vi "HardwareConfiguration.vi"() -> (3 "configured?":bool)   [LabVIEW 2019]
uses:
  InstrControl/InstrumentSetup.vi
  globals/QC_RunInformation.vi
  InstrControl/InstrControl.lvclass
panel:
  in  "Matrix Configurations":bool
  in  "Defaults Multimeter":bool
  in  "Multimeter":enum32{"Keithley 2000"}(tab)
  in  "Range Value\n(0.1 - 100)":dbl=100.0 format="%#.2g"
  in  "Range":u16(ring) items=["Auto", "Manual"]
  in  "Function":u16(ring)=3 items=["AC Current", "DC Current", "AC Voltage", "DC Voltage", "2W-Resistance", "4W-Resistance", "Period", "Frequency", "Temperature", "Diode", "Continuity"]
  in  "GPIB Address KE2000":refnum<visa-resource-name>
  in  "Defaults LCR":bool
  in  "LCRs":enum32{"WayneKerr 6440B", "WayneKerr 6425"}(tab)
  in  "AC frequency [Hz]":i32=1000 format="%#.3p"
  in  "RC Configuration":u16(ring) items=["serial", "parallel"]
  in  "AC amplitude [V]":sgl=0.1
  in  "GPIB Address WK6440B":refnum<visa-resource-name>
  in  "GPIB Address WK6425":refnum<visa-resource-name>
  in  "AC amplitude [V] WK6425":sgl=0.1 caption="AC amplitude [V]"
  in  "RC Configuration WK6425":u16(ring) caption="RC Configuration" items=["serial", "parallel"]
  in  "AC frequency [Hz] WK6425":i32=1000 caption="AC frequency [Hz]" format="%#.3p"
  in  "VISA address":refnum<visa-resource-name>="COM24" caption="Arduino address"
  out "Programm uploaded?":string="Make sure programme is uploaded to Arduino Uno ->"
  in  "Blank Button":bool
  in  "Supplies":T1(tab)
  in  "Current Limit [µA]":sgl=100.0
  in  "GPIB Address KE2410":refnum<visa-resource-name>
  in  "2657A Current Limit [µA]":sgl=100.0 caption="Current Limit [µA]"
  in  "GPIB Address 2657A":refnum<visa-resource-name>
  in  "GPIB Address KE487":refnum<visa-resource-name>
  in  "Compliance":u16(ring) items=["20µA", "2mA"]
  in  "Range:":u16(ring) items=["Autorange", "2nA", "20nA", "200nA", "2 microAmp", "20 microAmp", "200 microAmp", "2 milliAmp"]
  in  "Current Limit":u16(ring)=1 items=["OFF", "ON"]
  in  "GPIB Address KE6517":refnum<visa-resource-name>
  in  "current compliance \nlevel [mA]":dbl=0.0001 format="%.4f"
  in  "compliance/measurement\nrange (auto:0)":u16(ring)=6 items=["auto / auto", "1 nA / 1.1 V", "10 nA / 11 V", "100 nA / 110 V", "0.001 mA / 110 V", "0.01 mA / 110 V", "0.1 mA / 110 V", "1 mA / 110 V", "10 mA / 110 V", "100 mA / 110 V"]
  in  "GPIB Address KE236":refnum<visa-resource-name>
  in  "Defaults Supply":bool
  in  "OK Button":bool
  # "Hardware Configuration"
  # "Multimeter Configuration"
  # "Supply Configuration"
  # "Arduino Configuration"
  # "LCR Configuration"
  # "(Only for initialisation)"
  # "(Only for initialisation)"
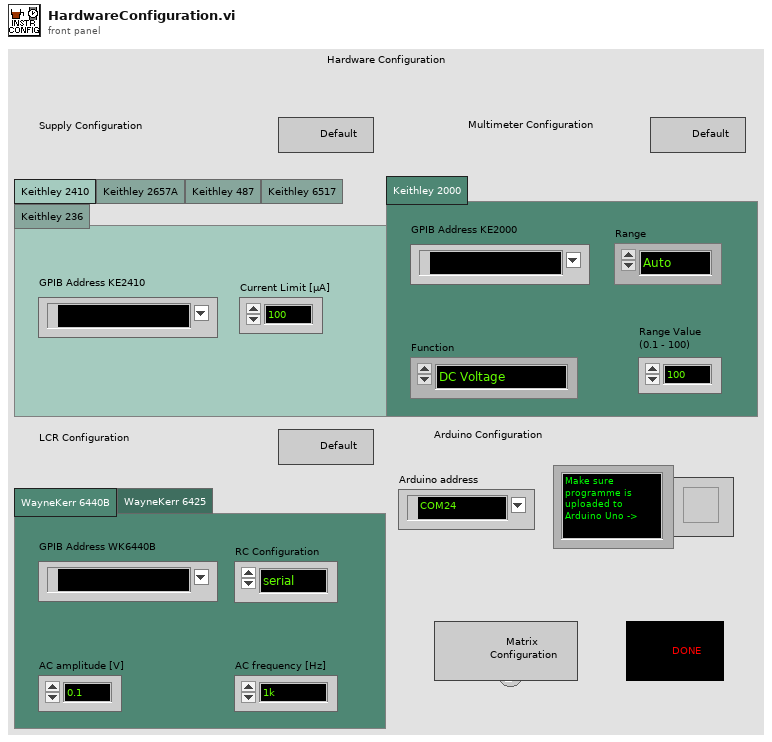
[diagram p1: front panel]
types:
  T1 = enum32{"Keithley 2410", "Keithley 2657A", "Keithley 487", "Keithley 6517", "Keithley 236"}
  T2 = cluster{"KE 2410":cluster{"Instrument name":string, "address":refnum<visa-resource-name>, "Instrument type":u16}, "KE 6517":cluster{"Instrument name":string, "address":refnum<visa-resource-name>, "Instrument type":u16}, "KE 487":cluster{"Instrument name":string, "address":refnum<visa-resource-name>, "Instrument type":u16}, "KE 236":cluster{"Instrument name":string, "address":refnum<visa-resource-name>, "Instrument type":u16}, "WK 6440B":cluster{"Instrument name":string, "address":refnum<visa-resource-name>, "Instrument type":u16}, "WK 6425":cluster{"Instrument name":string, "address":refnum<visa-resource-name>, "Instrument type":u16}, "Pickering Matrix":cluster{"Instrument name":string, "address":refnum<visa-resource-name>, "Instrument type":u16}, "KE 2000":cluster{"Instrument name":string, "address":refnum<visa-resource-name>, "Instrument type":u16}, "KE3706A Switching":cluster{"Instrument name":string, "address":refnum<visa-resource-name>, "Instrument type":u16}, "KE 2657A":cluster{"Instrument name":string, "address":refnum<visa-resource-name>, "Instrument type":u16}, "R_METAL KE2410":cluster{"Instrument name":string, "address":refnum<visa-resource-name>, "Instrument type":u16}, "HP34401A":cluster{"Instrument name":string, "address":refnum<visa-resource-name>, "Instrument type":u16}}
  T3 = cluster{"VISA address":refnum<visa-resource-name>, "T sensor":enum16{"SHT", "DS"}, "Arduino":refnum<class "ArduinoControl.lvclass">}
  T4 = cluster{"Range":u16, "Range Value":dbl, "Function":u16, "KE2000":refnum<class "KE2000.lvclass">}
  T5 = cluster{"Current Limit":sgl, "KE2410":refnum<class "KE2410.lvclass">}
  T6 = cluster{"Compliance":u16, "Range:":u16, "KE487":refnum<class "KE487.lvclass">}
  T7 = cluster{"Current Limit":sgl, "KE2657A":refnum<class "KE2657A.lvclass">}
  T8 = cluster{"Current Limit":u16, "KE6517":refnum<class "KE6517.lvclass">}
  T9 = cluster{"current \ncompliance level":dbl, "compliance/\nmeasurement range (auto:0)":u16, "KE236":refnum<class "KE236.lvclass">}
  T10 = cluster{"Sensor Serial No.:":string, "Wafer Serial No.:":string, "Batch:":string, "Manufacturer:":string, "Device Category:":string, "Database Serial No.:":string, "Date Initiated:":string, "Time Initiated:":string, "Test":string, "Instruments used:":string, "Probeplan used:":string, "End of Run comment:":string, "User:":string}
  T11 = cluster{"RC Configuration":u16, "AC amplitude [V]":dbl, "AC frequency [Hz]":i32, "WK6440B":refnum<class "WK6440B.lvclass">}
  T12 = cluster{"RC Configuration":u16, "AC amplitude [V]":dbl, "AC frequency [Hz]":i32, "WK6425":refnum<class "WK6425.lvclass">}
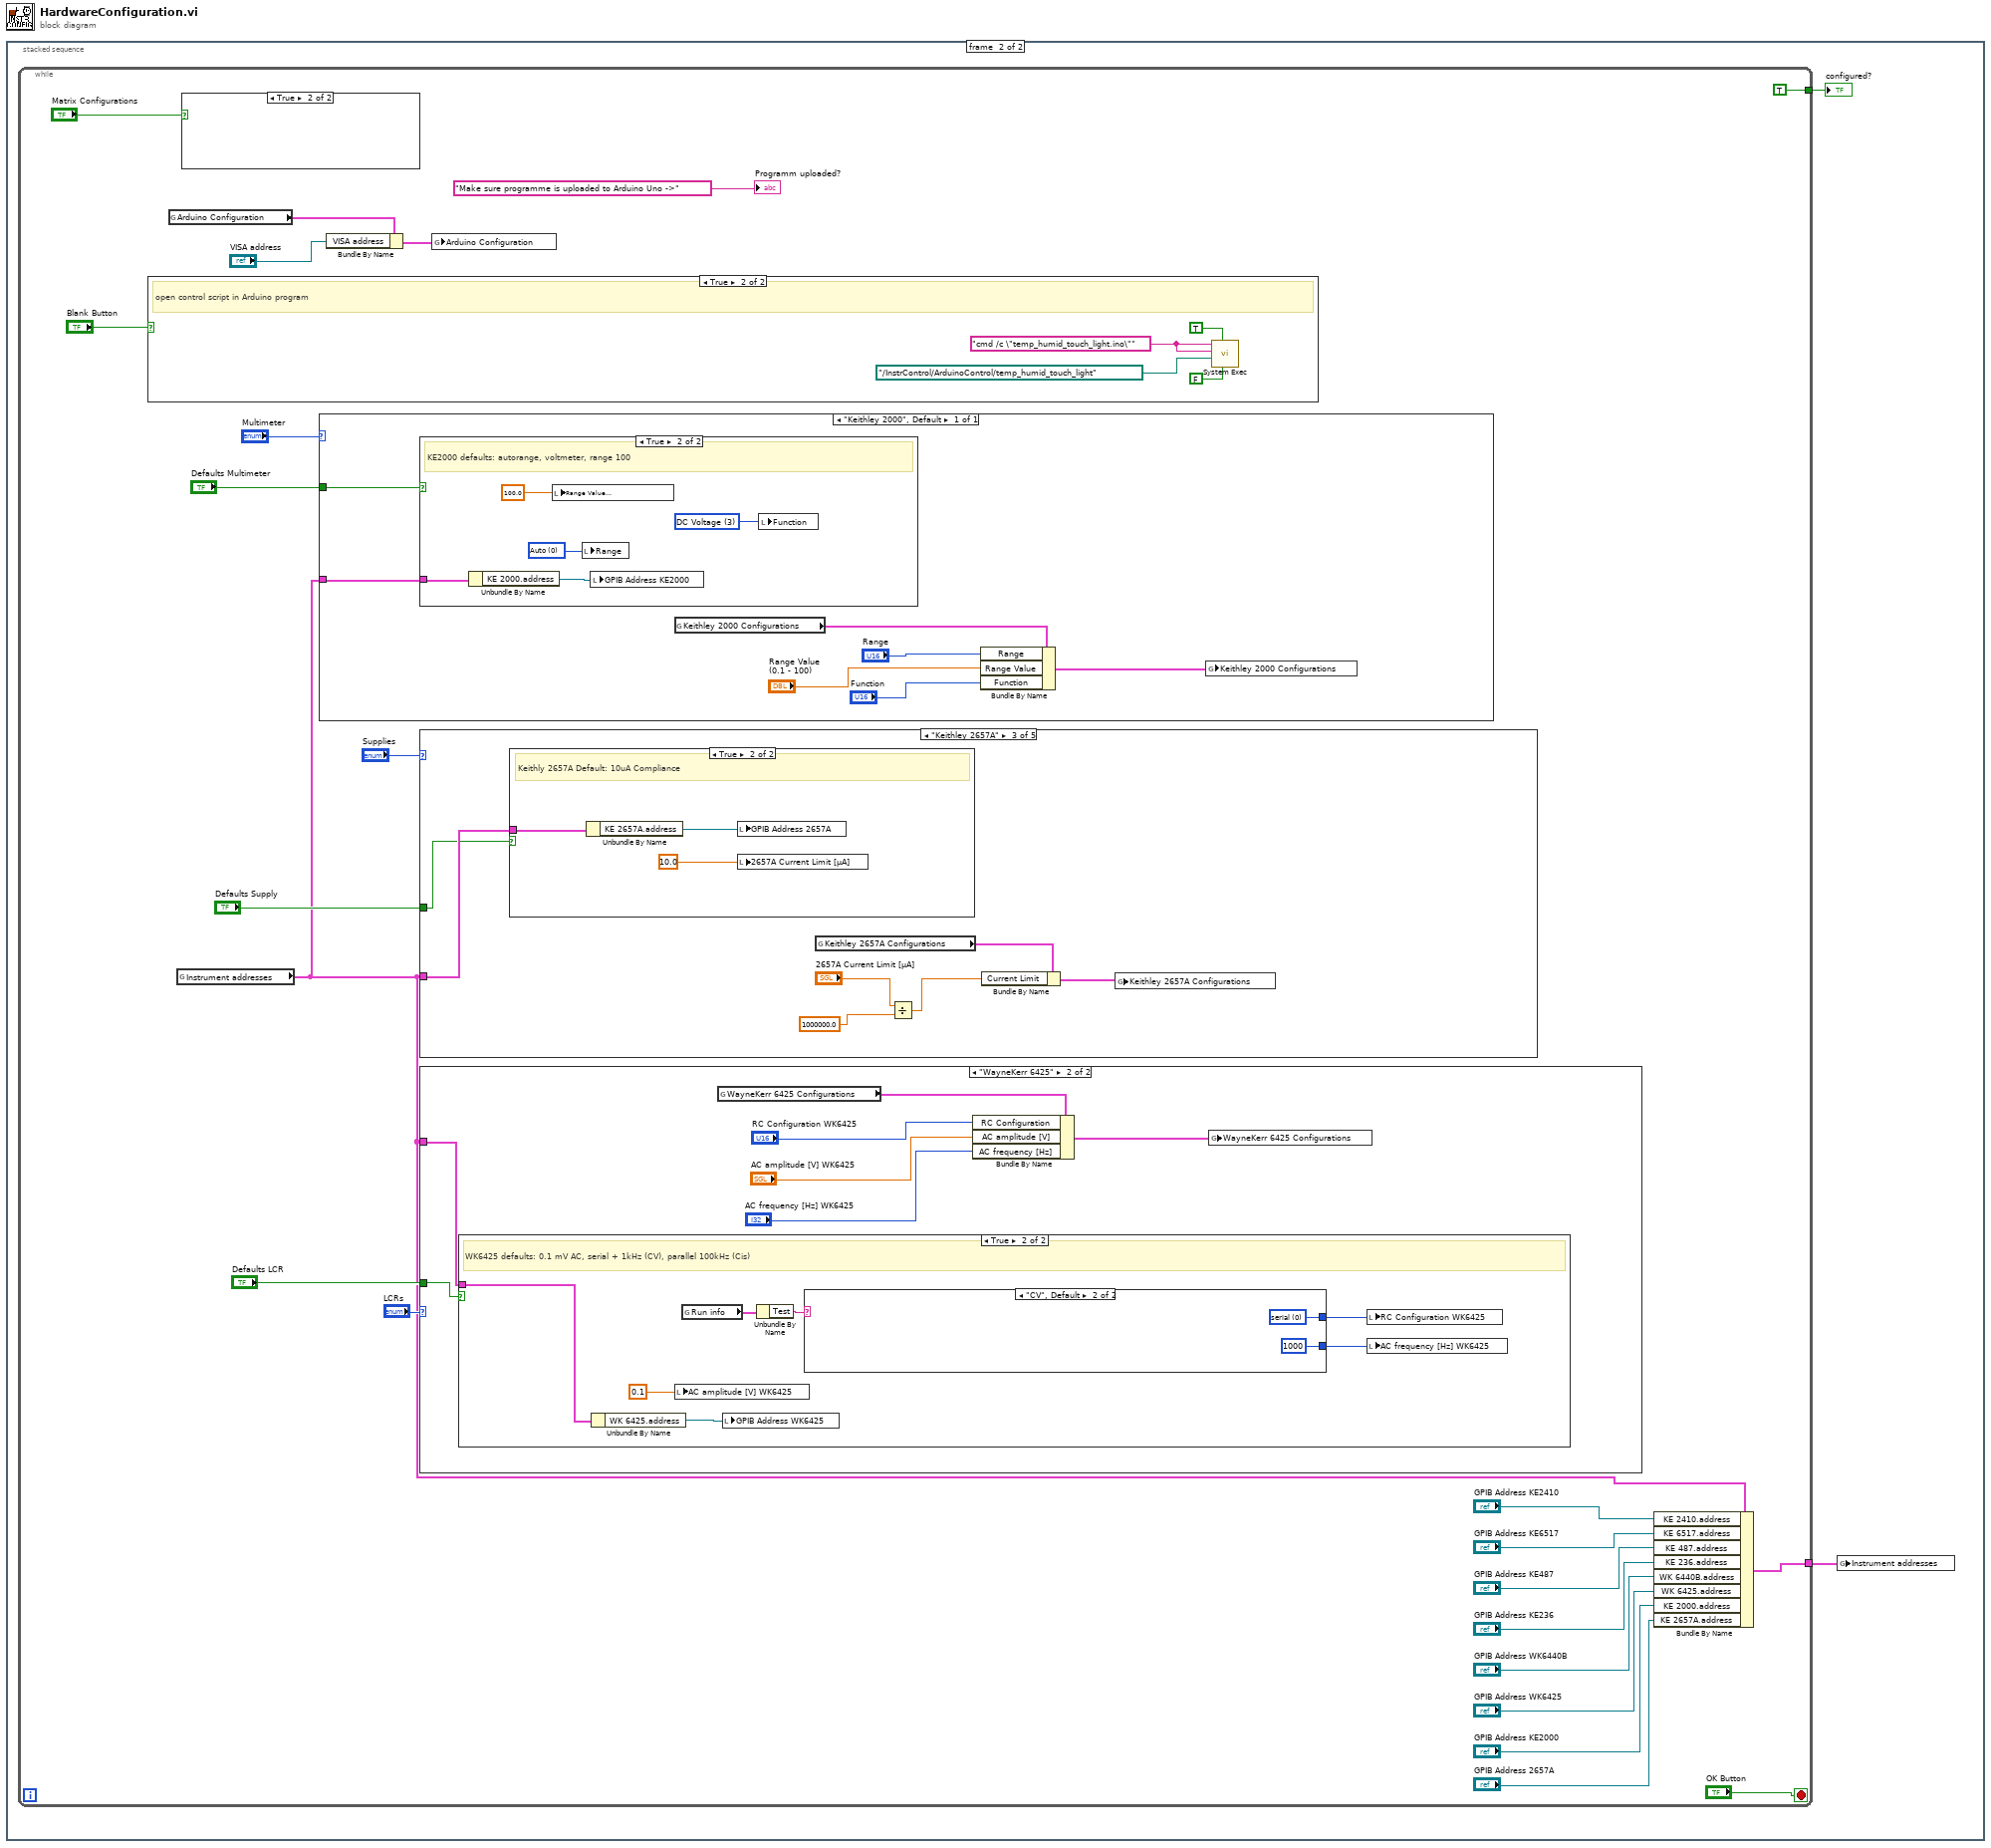
[diagram p0: block diagram]
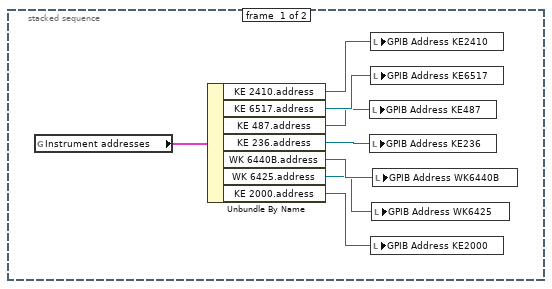
[diagram p2: hidden frame]
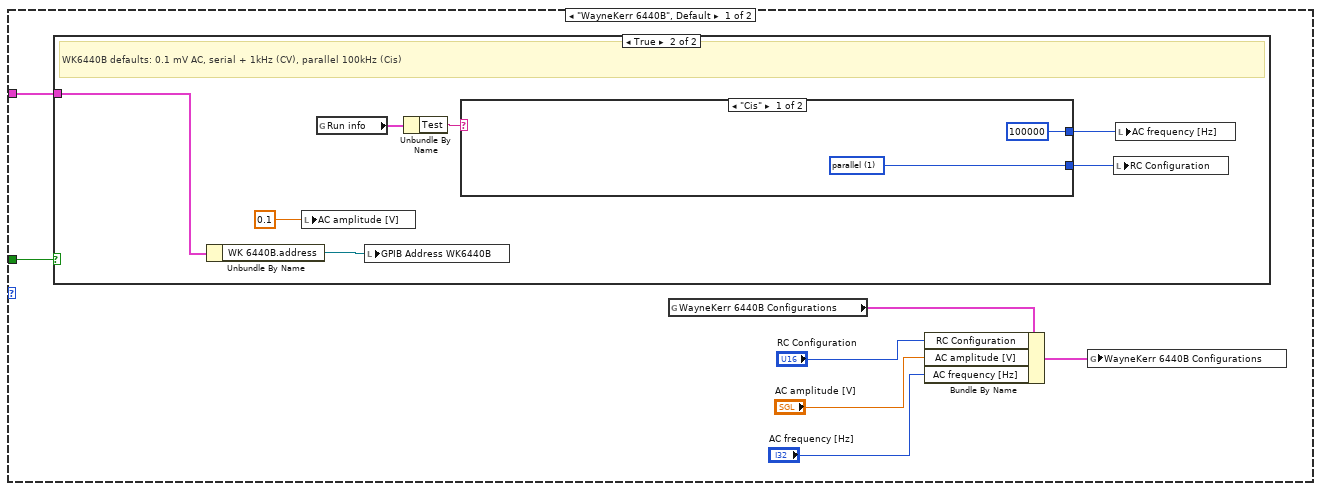
[diagram p6: hidden frame]
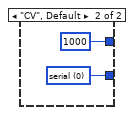
[diagram p8: hidden frame]
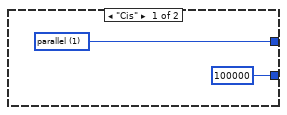
[diagram p10: hidden frame]
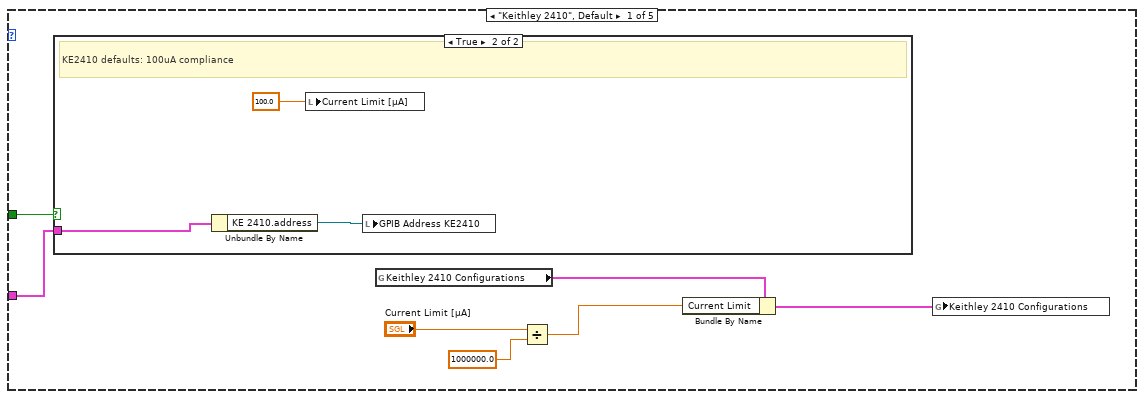
[diagram p11: hidden frame]
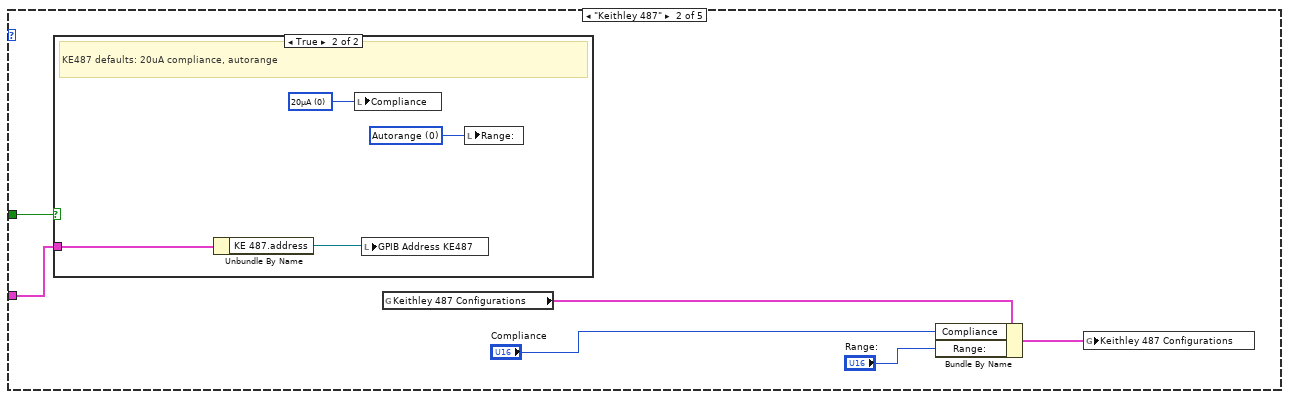
[diagram p13: hidden frame]
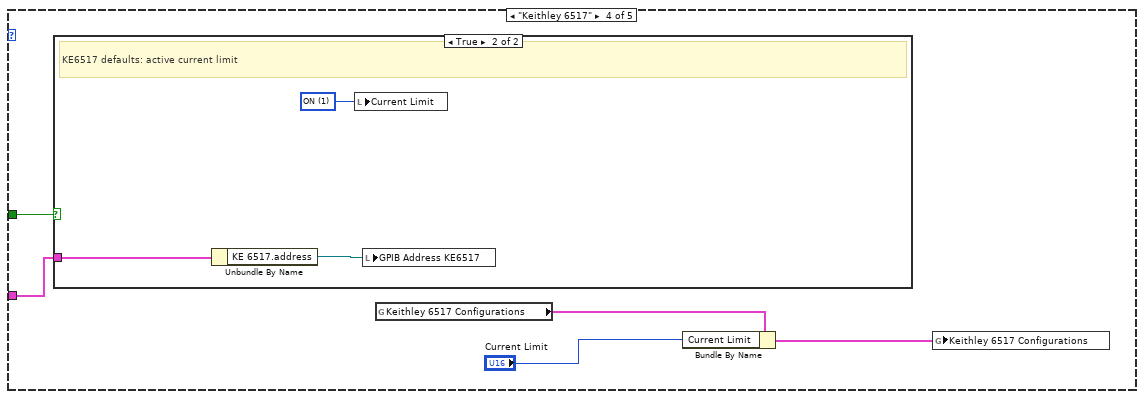
[diagram p16: hidden frame]
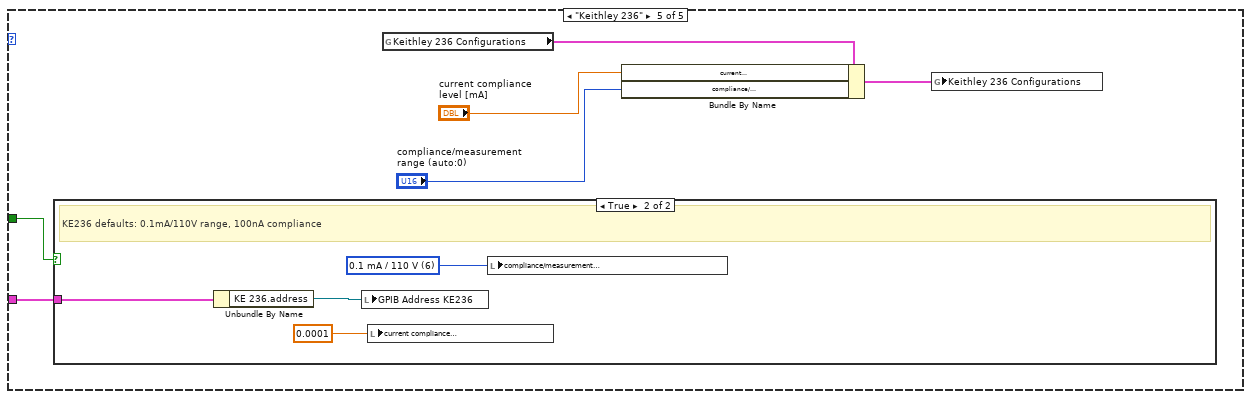
[diagram p18: hidden frame]
diagram:
  n1 = stacked-sequence {
    frame #0 {
      n2 = global read "InstrumentSetup.vi" "Instrument addresses"() -> (w8:T2)
      n3 = Unbundle By Name(w8) -> ("KE 2410.address"=w7:refnum<visa-resource-name>, "KE 6517.address"=w6:refnum<visa-resource-name>, "KE 487.address"=w5:refnum<visa-resource-name>, "KE 236.address"=w4:refnum<visa-resource-name>, "WK 6440B.address"=w3:refnum<visa-resource-name>, "WK 6425.address"=w2:refnum<visa-resource-name>, "KE 2000.address"=w1:refnum<visa-resource-name>)
      n4 = local write "GPIB Address KE487"(w5) -> ()
      n5 = local write "GPIB Address KE236"(w4) -> ()
      n6 = local write "GPIB Address KE2410"(w7) -> ()
      n7 = local write "GPIB Address KE6517"(w6) -> ()
      n8 = local write "GPIB Address KE2000"(w1) -> ()
      n9 = local write "GPIB Address WK6425"(w2) -> ()
      n10 = local write "GPIB Address WK6440B"(w3) -> ()
    }
    frame #1 {
      n11 = while {
        tunnel: [TRUE] -> w10
        tunnel: [w18] -> w9
        stop <- "OK Button" stop-if-true
        n12 = case shown="True" "Blank Button" {
          frame False {
          }
          frame True {
            w36 = "cmd /c \"temp_humid_touch_light.ino\""
            # "open control script in Arduino program"
            n13 = call <vilib>:"System Exec.vi"("run minimized? (F)"=FALSE, "wait until completion? (T)"=TRUE, "working directory"=path "../InstrControl/ArduinoControl/temp_humid_touch_light", "standard input"=w36, "command line"=w36) -> ()  [unwired: 3 in, 4 out]
          }
        }
        n14 = global read "InstrumentSetup.vi" "Arduino Configuration"() -> (w25:T3)
        n15 = global read "InstrumentSetup.vi" "Instrument addresses"() -> (w20:T2)
        n16 = case shown="True" "Matrix Configurations" {
          frame False {
          }
          frame True {
          }
        }
        n17 = case shown="\"Keithley 2000\", Default" "Multimeter" {
          tunnel: "Defaults Multimeter" -> [w45]
          tunnel: w20 -> [w42]
          frame "Keithley 2000", Default {
            n18 = case shown="True" w45 {
              tunnel: w42 -> [_ w50]
              frame False {
              }
              frame True {
                w48 = u16 0 items=["Auto", "Manual"] ("Range")
                w49 = u16 3 items=["AC Current", "DC Current", "AC Voltage", "DC Voltage", "2W-Resistance", "4W-Resistance", "Period", "Frequency", "Temperature", "Diode", "Continuity"] ("Function")
                # "KE2000 defaults: autorange, voltmeter, range 100"
                n19 = Unbundle By Name(w50) -> ("KE 2000.address"=w46:refnum<visa-resource-name>)
                n20 = local write "Range Value\n(0.1 - 100)"(100.0 ("Range Value\n(0.1 - 100)")) -> ()
                n21 = local write "Range"(w48) -> ()
                n22 = local write "GPIB Address KE2000"(w46) -> ()
                n23 = local write "Function"(w49) -> ()
              }
            }
            n24 = global read "InstrumentSetup.vi" "Keithley 2000 Configurations"() -> (w44:T4)
            n25 = Bundle By Name(cluster=w44, "Range"="Range", "Range Value"="Range Value\n(0.1 - 100)", "Function"="Function") -> (w43:T4)
            n26 = global write "InstrumentSetup.vi" "Keithley 2000 Configurations"(w43) -> ()
          }
        }
        n27 = Bundle By Name(cluster=w25, "VISA address"="VISA address") -> (w24:T3)
        n28 = case shown="\"Keithley 2657A\"" "Supplies" {
          tunnel: "Defaults Supply" -> [w93 w102 w112 w121 w130]
          tunnel: w20 -> [w88 w99 w113 w118 w127]
          frame "Keithley 2410", Default {
            n29 = case shown="True" w93 {
              tunnel: w88 -> [_ w96]
              frame False {
              }
              frame True {
                # "KE2410 defaults: 100uA compliance"
                n30 = Unbundle By Name(w96) -> ("KE 2410.address"=w94:refnum<visa-resource-name>)
                n31 = local write "Current Limit [µA]"(100.0) -> ()
                n32 = local write "GPIB Address KE2410"(w94) -> ()
              }
            }
            n33 = global read "InstrumentSetup.vi" "Keithley 2410 Configurations"() -> (w92:T5)
            n34 = Divide(x="Current Limit [µA]", y=1000000.0) -> (x/y=w89:dbl)
            n35 = Bundle By Name(cluster=w92, "Current Limit"=w89) -> (w91:T5)
            n36 = global write "InstrumentSetup.vi" "Keithley 2410 Configurations"(w91) -> ()
          }
          frame "Keithley 487" {
            n37 = case shown="True" w102 {
              tunnel: w99 -> [_ w106]
              frame False {
              }
              frame True {
                w104 = u16 0 items=["Autorange", "2nA", "20nA", "200nA", "2 microAmp", "20 microAmp", "200 microAmp", "2 milliAmp"] ("Range:")
                w105 = u16 0 items=["20µA", "2mA"] ("Compliance")
                # "KE487 defaults: 20uA compliance, autorange"
                n38 = Unbundle By Name(w106) -> ("KE 487.address"=w103:refnum<visa-resource-name>)
                n39 = local write "Compliance"(w105) -> ()
                n40 = local write "GPIB Address KE487"(w103) -> ()
                n41 = local write "Range:"(w104) -> ()
              }
            }
            n42 = global read "InstrumentSetup.vi" "Keithley 487 Configurations"() -> (w101:T6)
            n43 = Bundle By Name(cluster=w101, "Compliance"="Compliance", "Range:"="Range:") -> (w100:T6)
            n44 = global write "InstrumentSetup.vi" "Keithley 487 Configurations"(w100) -> ()
          }
          frame "Keithley 2657A" {
            n45 = case shown="True" w112 {
              tunnel: w113 -> [_ w116]
              frame False {
              }
              frame True {
                # "Keithly 2657A Default: 10uA Compliance"
                n46 = Unbundle By Name(w116) -> ("KE 2657A.address"=w115:refnum<visa-resource-name>)
                n47 = local write "GPIB Address 2657A"(w115) -> ()
                n48 = local write "2657A Current Limit [µA]"(sgl 10.0 ("2657A Current Limit [µA]")) -> ()
              }
            }
            n49 = global read "InstrumentSetup.vi" "Keithley 2657A Configurations"() -> (w111:T7)
            n50 = Divide(x="2657A Current Limit [µA]", y=1000000.0) -> (x/y=w109:dbl)
            n51 = Bundle By Name(cluster=w111, "Current Limit"=w109) -> (w110:T7)
            n52 = global write "InstrumentSetup.vi" "Keithley 2657A Configurations"(w110) -> ()
          }
          frame "Keithley 6517" {
            n53 = case shown="True" w121 {
              tunnel: w118 -> [_ w124]
              frame False {
              }
              frame True {
                w123 = u16 1 items=["OFF", "ON"] ("Current Limit")
                # "KE6517 defaults: active current limit"
                n54 = Unbundle By Name(w124) -> ("KE 6517.address"=w122:refnum<visa-resource-name>)
                n55 = local write "Current Limit"(w123) -> ()
                n56 = local write "GPIB Address KE6517"(w122) -> ()
              }
            }
            n57 = global read "InstrumentSetup.vi" "Keithley 6517 Configurations"() -> (w120:T8)
            n58 = Bundle By Name(cluster=w120, "Current Limit"="Current Limit") -> (w119:T8)
            n59 = global write "InstrumentSetup.vi" "Keithley 6517 Configurations"(w119) -> ()
          }
          frame "Keithley 236" {
            n60 = case shown="True" w130 {
              tunnel: w127 -> [_ w134]
              frame False {
              }
              frame True {
                w132 = u16 6 items=["auto / auto", "1 nA / 1.1 V", "10 nA / 11 V", "100 nA / 110 V", "0.001 mA / 110 V", "0.01 mA / 110 V", "0.1 mA / 110 V", "1 mA / 110 V", "10 mA / 110 V", "100 mA / 110 V"] ("compliance/\nmeasurement range (auto:0)")
                # "KE236 defaults: 0.1mA/110V range, 100nA compliance"
                n61 = Unbundle By Name(w134) -> ("KE 236.address"=w131:refnum<visa-resource-name>)
                n62 = local write "GPIB Address KE236"(w131) -> ()
                n63 = local write "current compliance \nlevel [mA]"(0.0001 ("current \ncompliance level")) -> ()
                n64 = local write "compliance/measurement\nrange (auto:0)"(w132) -> ()
              }
            }
            n65 = global read "InstrumentSetup.vi" "Keithley 236 Configurations"() -> (w128:T9)
            n66 = Bundle By Name(cluster=w128, "current \ncompliance level"="current compliance \nlevel [mA]", "compliance/\nmeasurement range (auto:0)"="compliance/measurement\nrange (auto:0)") -> (w129:T9)
            n67 = global write "InstrumentSetup.vi" "Keithley 236 Configurations"(w129) -> ()
          }
        }
        n68 = case shown="\"WayneKerr 6425\"" "LCRs" {
          tunnel: "Defaults LCR" -> [w55 w73]
          tunnel: w20 -> [w54 w72]
          frame "WayneKerr 6440B", Default {
            n69 = case shown="True" w55 {
              tunnel: w54 -> [_ w64]
              frame False {
              }
              frame True {
                # "WK6440B defaults: 0.1 mV AC, serial + 1kHz (CV), parallel 100kHz (Cis)"
                n70 = Unbundle By Name(w64) -> ("WK 6440B.address"=w58:refnum<visa-resource-name>)
                n71 = local write "AC amplitude [V]"(0.1) -> ()
                n72 = global read "QC_RunInformation.vi" "Run info"() -> (w60:T10)
                n73 = local write "GPIB Address WK6440B"(w58) -> ()
                n74 = Unbundle By Name(w60) -> ("Test"=w59:string)
                n75 = case shown="\"Cis\"" w59 {
                  tunnel: [w66 w68] -> w62
                  tunnel: [100000 1000] -> w61
                  frame "Cis" {
                    w66 = u16 1 items=["serial", "parallel"] ("RC Configuration")
                  }
                  frame "CV", Default {
                    w68 = u16 0 items=["serial", "parallel"] ("RC Configuration")
                  }
                }
                n76 = local write "RC Configuration"(w62) -> ()
                n77 = local write "AC frequency [Hz]"(w61) -> ()
              }
            }
            n78 = global read "InstrumentSetup.vi" "WayneKerr 6440B Configurations"() -> (w57:T11)
            n79 = Bundle By Name(cluster=w57, "RC Configuration"="RC Configuration", "AC amplitude [V]"="AC amplitude [V]", "AC frequency [Hz]"="AC frequency [Hz]") -> (w56:T11)
            n80 = global write "InstrumentSetup.vi" "WayneKerr 6440B Configurations"(w56) -> ()
          }
          frame "WayneKerr 6425" {
            n81 = case shown="True" w73 {
              tunnel: w72 -> [_ w82]
              frame False {
              }
              frame True {
                # "WK6425 defaults: 0.1 mV AC, serial + 1kHz (CV), parallel 100kHz (Cis)"
                n82 = Unbundle By Name(w82) -> ("WK 6425.address"=w76:refnum<visa-resource-name>)
                n83 = local write "AC amplitude [V] WK6425"(0.1) -> ()
                n84 = global read "QC_RunInformation.vi" "Run info"() -> (w78:T10)
                n85 = local write "GPIB Address WK6425"(w76) -> ()
                n86 = Unbundle By Name(w78) -> ("Test"=w77:string)
                n87 = case shown="\"CV\", Default" w77 {
                  tunnel: [w84 w86] -> w80
                  tunnel: [100000 1000] -> w79
                  frame "Cis" {
                    w84 = u16 1 items=["serial", "parallel"] ("RC Configuration")
                  }
                  frame "CV", Default {
                    w86 = u16 0 items=["serial", "parallel"] ("RC Configuration")
                  }
                }
                n88 = local write "RC Configuration WK6425"(w80) -> ()
                n89 = local write "AC frequency [Hz] WK6425"(w79) -> ()
              }
            }
            n90 = global read "InstrumentSetup.vi" "WayneKerr 6425 Configurations"() -> (w75:T12)
            n91 = Bundle By Name(cluster=w75, "RC Configuration"="RC Configuration WK6425", "AC amplitude [V]"="AC amplitude [V] WK6425", "AC frequency [Hz]"="AC frequency [Hz] WK6425") -> (w74:T12)
            n92 = global write "InstrumentSetup.vi" "WayneKerr 6425 Configurations"(w74) -> ()
          }
        }
        n93 = global write "InstrumentSetup.vi" "Arduino Configuration"(w24) -> ()
        n94 = Bundle By Name(cluster=w20, "KE 2410.address"="GPIB Address KE2410", "KE 6517.address"="GPIB Address KE6517", "KE 487.address"="GPIB Address KE487", "KE 236.address"="GPIB Address KE236", "WK 6440B.address"="GPIB Address WK6440B", "WK 6425.address"="GPIB Address WK6425", "KE 2000.address"="GPIB Address KE2000", "KE 2657A.address"="GPIB Address 2657A") -> (w18:T2)
        "Programm uploaded?" <- "Make sure programme is uploaded to Arduino Uno ->"
      }
      "configured?" <- w10
      n95 = global write "InstrumentSetup.vi" "Instrument addresses"(w9) -> ()
    }
  }
